vi "Update Check-in Status.vi"(0 "Hotel Management Tool Model in":refnum<class "Hotel Management Tool Model.lvclass">, 5 "Rooms Manager GUID":string, 7 "IsSuccess":bool, 9 "Room No":string, 11 "error in (no error)":errorcluster, 12 "Reason If Failure":string) -> (4 "Hotel Management Tool Model out":refnum<class "Hotel Management Tool Model.lvclass">, 15 "error out":errorcluster)   [LabVIEW 2023, in "Hotel Management Tool Model.lvlib" / "Hotel Management Tool Model.lvclass"]
uses:
  Hotel Management Tool Model.lvclass
  Hotel Management Tool Model.lvclass/Hotel Management Tool Model.ctl
  Rooms Manager Model/Rooms Manager Model Messages/Update Check-in Status Msg/Update Check-in Status Msg.lvclass/Update Check-in Status Msg.ctl
  <vilib>/ActorFramework/Message Enqueuer/Message Enqueuer.lvclass/Message Enqueuer.ctl
  <vilib>/ActorFramework/Message Enqueuer/Enqueue.vi
  Rooms Manager Model/Rooms Manager Model Messages/Update Check-in Status Msg/Update Check-in Status Msg.lvclass
  C:/Program Files/National Instruments/LabVIEW 2023/vi.lib/ActorFramework/Message/Message.lvclass
  <vilib>/ActorFramework/Message Priority Queue/Priority Enqueue.vi
  <vilib>/ActorFramework/Actor/Actor.lvclass
  Room Service Manager Model/Room Service Manager Model/Room Service Manager Model.lvclass
  Room Service Manager Model/Room Service Manager Model Messages/Update Title Msg/Update Title Msg.lvclass
  C:/Users/bhaghyaraj/Trainings/NI Actor Framework/SDLC/Model Base/Model Base/Model Base.lvclass
  C:/Program Files/National Instruments/LabVIEW 2023/vi.lib/ActorFramework/Actor/Actor.lvclass
  C:/Users/bhaghyaraj/Trainings/NI Actor Framework/SDLC/Interfaces/Model Base/Incoming Model Base Interface.lvclass
  C:/Users/bhaghyaraj/Trainings/NI Actor Framework/SDLC/Room Service Manager Model/Room Service Manager Model/Room Service Manager Model.lvclass
  C:/Users/bhaghyaraj/Trainings/NI Actor Framework/SDLC/Hotel Management Tool Model/Hotel Management Tool Model/Hotel Management Tool Model.lvclass
  C:/Users/bhaghyaraj/Trainings/NI Actor Framework/SDLC/Interfaces/Hotel Management Tool Model/Incoming Hotel Management Tool Model Interface.lvclass
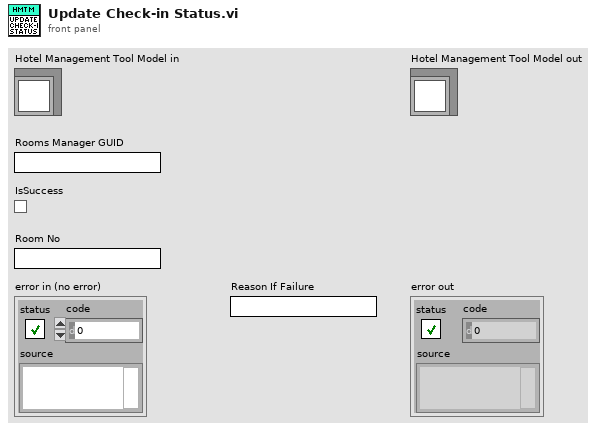
[diagram p1: front panel]
types:
  T1 = map{string, refnum<class "Message Enqueuer.lvclass">}
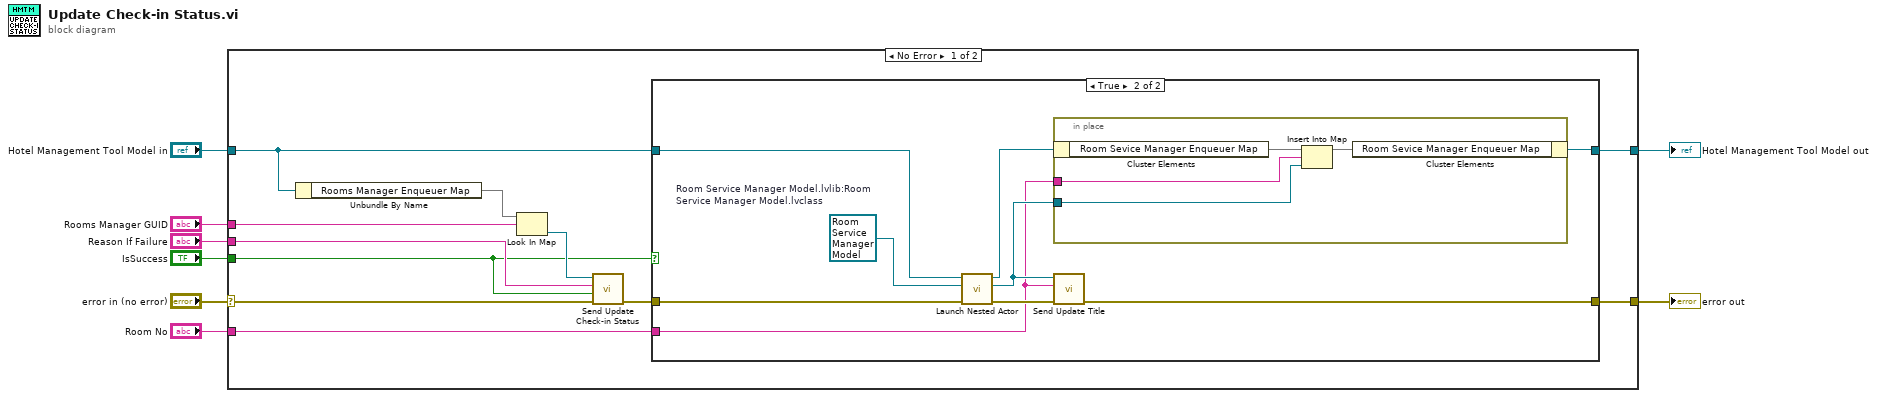
[diagram p0: block diagram]
diagram:
  n1 = case shown="No Error" "error in (no error)" {
    selector: "error in (no error)" -> [w19 w36]
    tunnel: [w13 w36] -> w7
    tunnel: "Hotel Management Tool Model in" -> [w12 w35]
    tunnel: "Rooms Manager GUID" -> [w16 _]
    tunnel: "Reason If Failure" -> [w15 _]
    tunnel: "IsSuccess" -> [w11 _]
    tunnel: [w9 w35] -> w2
    tunnel: "Room No" -> [w10 _]
    frame No Error {
      n2 = Unbundle By Name(w12) -> ("Rooms Manager Enqueuer Map"=w17:T1)
      n3 = Look In Map(map=w17, key=w16) -> (value=w14:refnum<class "Message Enqueuer.lvclass">)  [unwired: 1 in, 1 out]
      n4 = call "Send Update Check-in Status.vi"("error in (no error)"=w19, "IsSuccess"=w11, "Reason If Failure"=w15, "Message Enqueuer"=w14) -> ("error out"=w18:errorcluster)  [unwired: 6 in, 1 out]
      n5 = case shown="True" w11 {
        tunnel: w18 -> [w20 w30]
        tunnel: [w20 w26] -> w13
        tunnel: w12 -> [w21 w28]
        tunnel: w10 -> [_ w22]
        tunnel: [w21 w24] -> w9
        frame False {
        }
        frame True {
          w27 = refnum<class "Room Service Manager Model.lvclass"> refnum  # Room Service Manager Model.lvlib:Room Service Manager Model.lvclass
          n6 = call <vilib>:"Launch Nested Actor.vi"("error in (no error)"=w30, "Nested Actor"=w27, "Caller Actor in"=w28) -> ("error out"=w29:errorcluster, "Nested Actor's Enqueuer"=w23:refnum<class "Message Enqueuer.lvclass">, "Caller Actor out"=w25:refnum<class "Hotel Management Tool Model.lvclass">)  [unwired: 6 in]
          n7 = in-place {
            in-place-border: w23 -> [w32]
            in-place-border: w22 -> [w31]
            n8 = in-place-cluster #1(w25) -> ("Room Sevice Manager Enqueuer Map"=w34:T1)
            n9 = Insert Into Map(map in=w34, key=w31, value=w32) -> (map out=w33:T1)  [unwired: 2 out]
            n10 = in-place-cluster #1("Room Sevice Manager Enqueuer Map"=w33) -> (w24:refnum<class "Hotel Management Tool Model.lvclass">)
          }
          n11 = call "Send Update Title.vi"("error in (no error)"=w29, "Room No"=w22, "Message Enqueuer"=w23) -> ("error out"=w26:errorcluster)  [unwired: 7 in, 1 out]
        }
      }
    }
    frame Error {
    }
  }
  "error out" <- w7
  "Hotel Management Tool Model out" <- w2
